vi "Get Attribute DBL.vi"(8 "error in":errorcluster, 10 "Attribute":string, 11 "ConfigFromJSON in":refnum<class "Config from JSON.lvclass">) -> (0 "error out":errorcluster, 2 "Value":dbl, 3 "ConfigFromJSON out":refnum<class "Config from JSON.lvclass">)   [LabVIEW 2025, in "Config from JSON.lvclass"]
uses:
  Config from JSON.lvclass
  Config from JSON.lvclass/Config from JSON.ctl
  f81bb2d8-f854-41c0-af1a-a658860601c6.vi
  f81bb2d8-f854-41c0-af1a-a658860601c6.vi/a4169a97-72fc-4003-a778-603cf20cafa0.vi
  <vilib>/Utility/error.llb/Trim Whitespace.vi
  <vilib>/JDP Science/JSONtext/Find Item.vi
  <vilib>/Utility/error.llb/Trim Whitespace One-Sided.vi
  <vilib>/JDP Science/JSONtext/Next JSON Value.vi
  <vilib>/JDP Science/JSONtext/String Subset.vi
  <vilib>/JDP Science/JSONtext/Parsing/Advance past next JSON Value (inlined COPY).vi
  <vilib>/JDP Science/JSONtext/Parsing/Advance past whitespace.vi
  <vilib>/JDP Science/JSONtext/Parsing/Advance past String.vi
  <vilib>/JDP Science/JSONtext/Parsing/Advance past Number.vi
  <vilib>/JDP Science/JSONtext/Parsing/Advance past Line Ending.vi
  <vilib>/JDP Science/JSONtext/Parsing/Parse Full Path or Item Name.vi
  <vilib>/JDP Science/JSONtext/Parsing/Advance past Array.vi
  <vilib>/JDP Science/JSONtext/Parsing/Advance past Object.vi
  <vilib>/JDP Science/JSONtext/support/Error Cluster From Code.vi
  <vilib>/JDP Science/JSONtext/Offset/Find Item Locations by Path.vi
  <vilib>/JDP Science/JSONtext/JSON text to Variant.vi
  Common-LabVIEW-Helpers/Source/errors/-8301 Item not found in JSON--error.vi
  Common-LabVIEW-Helpers/Source/errors/-8300 JSON empty--error.vi
  <vilib>/JDP Science/JSONtext/LVClass Serializer/JSONtext LVClass Serializer.lvclass
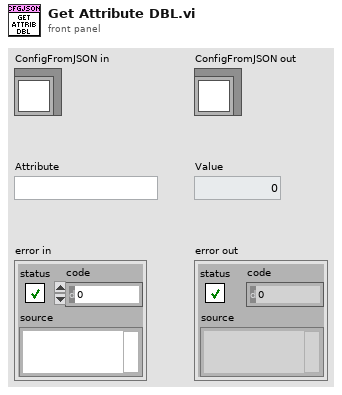
[diagram p1: front panel]
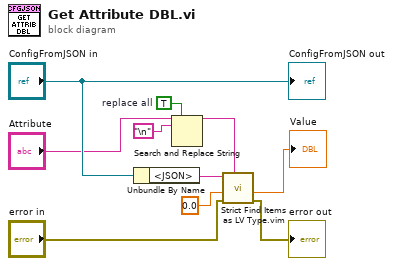
[diagram p0: block diagram]
diagram:
  w1 = TRUE  # replace all
  n1 = Unbundle By Name("ConfigFromJSON in") -> ("<JSON>"=w9:string)
  n2 = Search and Replace String(replace all?=w1, input string="Attribute", search string="\n") -> (result string=w2:string)  [unwired: 5 in, 3 out]
  n3 = call "Strict Find Items as LV Type.vim"("$Path or Item Name"=w2, "error in"="error in", "Data Type and Default Value"=0.0, "<JSON>"=w9) -> ("error out"=→"error out":errorcluster, "Data out"=→"Value":dbl)  [unwired: 5 in, 1 out]
  "ConfigFromJSON out" <- "ConfigFromJSON in"
